vi "Delete_Variant.vi"(8 "error in (no error)":errorcluster, 10 "Delete variant":string, 11 "configuration file path":path) -> (0 "error out":errorcluster, 3 "file path":path)   [LabVIEW 2021]
uses:
  <vilib>/Utility/config.llb/NI_LVConfig.lvlib
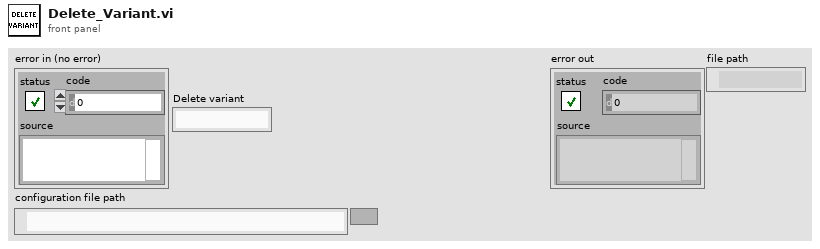
[diagram p1: front panel]
types:
  T1 = typedef "NI_LVConfig.lvlib/Config Data RefNum.ctl" = refnum<k1>
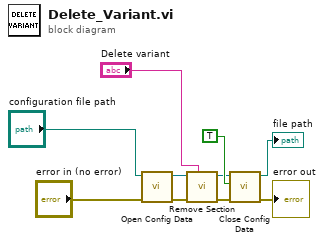
[diagram p0: block diagram]
diagram:
  n1 = call <vilib>:"Open Config Data.vi"("error in (no error)"="error in (no error)", "configuration file path"="configuration file path") -> ("error out"=w1:errorcluster, "refnum"=w2:T1)  [unwired: 7 in, 1 out]
  n2 = call <vilib>:"Remove Section.vi"("section"="Delete variant", "error in (no error)"=w1, "refnum"=w2) -> ("error out"=w4:errorcluster, "refnum out"=w5:T1)  [unwired: 6 in, 1 out]
  n3 = call <vilib>:"Close Config Data.vi"("error in (no error)"=w4, "write file if changed (T)"=TRUE, "refnum"=w5) -> ("error out"=→"error out":errorcluster, "file path"=→"file path":path)  [unwired: 7 in]
